vi "PID control.vi"(4 "auto? (F)":bool, 5 "dt (s)":dbl, 6 "PID gains":T1={"proportional gain (Kc)"=1.0, "integral time (Ti, min)"=0.01, "derivative time (Td, min)"=0.0} {"derivative time (Td, min)" format="%#.6g"; "integral time (Ti, min)" format="%#.6g"; "proportional gain (Kc)" format="%#.6g"}, 7 "Waveform Function (0: Sine)":u16(ring)=1 items=["Sine", "Square", "Ramp", "DC", "Pulse", "Arb"], 8 "error in (no error)":errorcluster, 9 "Frequency (Hz)":dbl=1000.0 min=1e-06 max=160000000.0 step=1.0 format="%#.6g", 10 "Amplitude setpoint (V)":dbl=1.0 min=0.001 max=20.0 step=1.0 format="%#.3f", 11 "VISA resource name":refnum<visa-resource-name>) -> (0 "error out":errorcluster, 3 "VISA resource name out":refnum<visa-resource-name>)   [LabVIEW 2017]
uses:
  <vilib>/addons/control/pid/autopid.llb/PID autotuning parameters (adv).ctl
  <vilib>/DAQmx/read.llb/DAQmx Read (Analog Wfm 1Chan NSamp).vi
  <vilib>/Analysis/baseanly.llb/Mean (DBL).vi
  <vilib>/DAQmx/miscellaneous.llb/DAQmx Fill In Error Info.vi
  <instrlib>/Siglent SDG 1000 5000 800 Series/Siglent SDG 1000 5000 800 Series.lvlib
  <vilib>/Analysis/NI_AALBase.lvlib
  <vilib>/addons/control/pid/NI_PID_autopid.lvlib
panel:
  in  "stop":bool
  out "Measured amplitude (V)":dbl format="%0.2f"
  out "tuning completed?":bool
  out "Control amplitude (V)":dbl
  in  "output range":cluster{"output high":dbl, "output low":dbl}={"output high"=10.0, "output low"=0.0}
  out "tuned PID gains":T1={"proportional gain (Kc)"=1.0, "integral time (Ti, min)"=0.01, "derivative time (Td, min)"=0.0} {"derivative time (Td, min)" format="%#.6g"; "integral time (Ti, min)" format="%#.6g"; "proportional gain (Kc)" format="%#.6g"}
  in  "autotuning parameters":T2={"technique"=2, "type of controller"=1, "control specification"=0, "amplitude"=1.0} {"amplitude" format="%.2f"; "control specification" items=["normal", "fast", "slow"]; "type of controller" items=["P", "PI", "PID"]; "technique" items=["Step Open Loop", "Step Closed Loop", "Relay", "PID Relay"]}
  in  "reinitialize? (F)":bool
  in  "autotune? (F)":bool
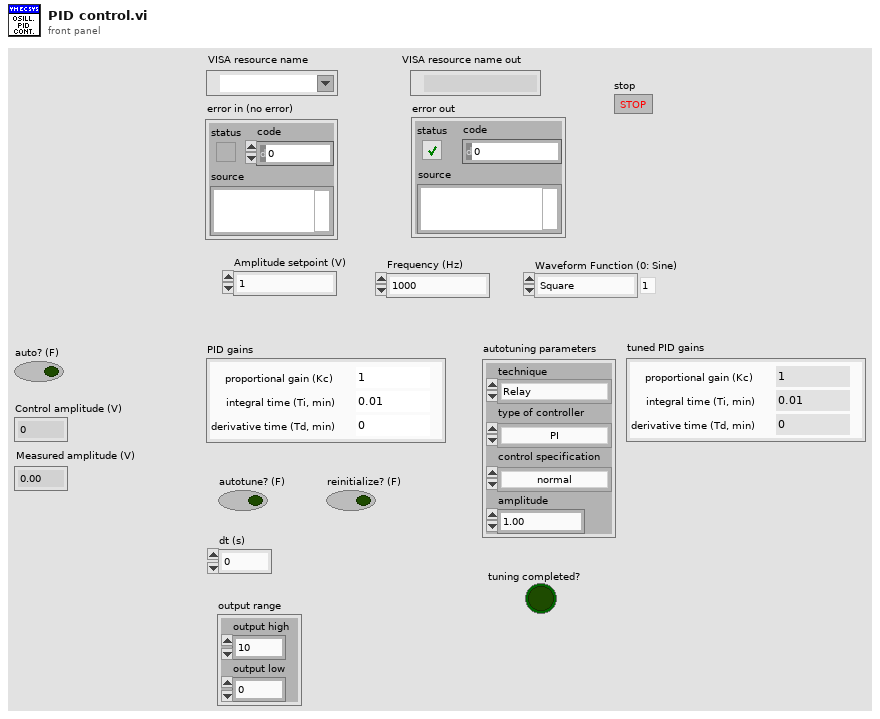
[diagram p1: front panel]
types:
  T1 = cluster{"proportional gain (Kc)":dbl, "integral time (Ti, min)":dbl, "derivative time (Td, min)":dbl}
  T2 = typedef "NI_PID_autopid.lvlib/PID autotuning parameters (adv).ctl" = cluster{"technique":u16, "type of controller":u16, "control specification":u16, "amplitude":dbl}
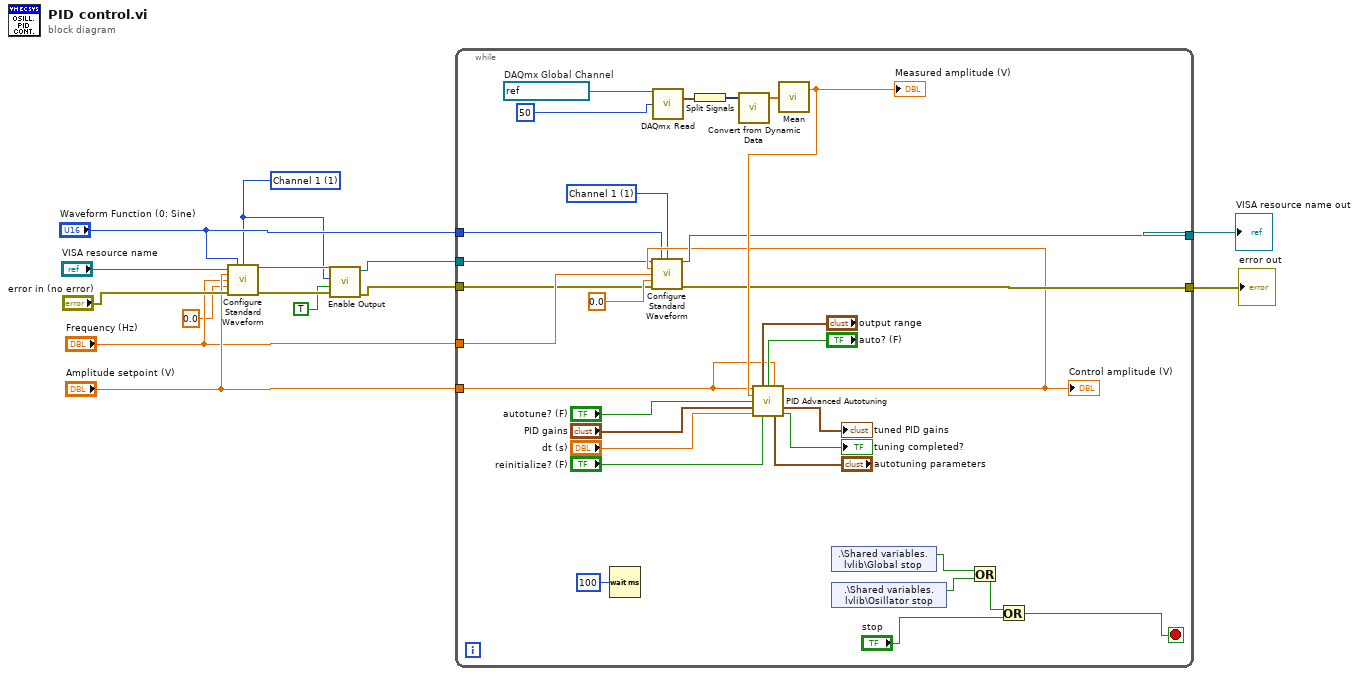
[diagram p0: block diagram]
diagram:
  w2 = 1 items=["Channel 1"=1, "Channel 2"=2] ("Channel (1:Channel 1)")
  n1 = call <instrlib>:"Configure Standard Waveform.vi"("VISA resource name"="VISA resource name", "Waveform Function (0: Sine)"="Waveform Function (0: Sine)", "Channel (1:Channel 1)"=w2, "Amplitude (1.0 Vpp)"="Amplitude setpoint (V)", "Frequency (1000 Hz)"="Frequency (Hz)", "DC Offset (0.00 V)"=0.0, "error in (no error)"="error in (no error)") -> ("VISA resource name out"=w9:refnum<visa-resource-name>, "error out"=w10:errorcluster)  [unwired: 7 in]
  n2 = call <instrlib>:"Enable Output.vi"("error in (no error)"=w10, "Enable Output (T: Enable)"=TRUE, "Channel (1:Channel 1)"=w2, "VISA resource name"=w9) -> ("error out"=w7:errorcluster, "VISA resource name out"=w8:refnum<visa-resource-name>)  [unwired: 6 in]
  n3 = while {
    tunnel: "Frequency (Hz)" -> [w40]
    tunnel: "Amplitude setpoint (V)" -> [w25]
    tunnel: [w31] -> w14
    tunnel: [w30] -> w13
    tunnel: "Waveform Function (0: Sine)" -> [w18]
    tunnel: w8 -> [w17]
    tunnel: w7 -> [w16]
    stop <- w19 stop-if-true
    w15 = 1 items=["Channel 1"=1, "Channel 2"=2] ("Channel (1:Channel 1)")
    w45 = refnum<k21> "AC voltage"  # DAQmx Global Channel
    n4 = Wait (ms)(milliseconds to wait=u32 100) -> ()  [unwired: 1 out]
    n5 = call-poly <vilib>:"DAQmx Read.vi"("task/channels in"=w45, "number of samples per channel"=50) -> ("data"=w44:waveform(dbl))  [unwired: 11 in, 2 out]
    n6 = Split Signals(w44) -> (w43:dynamicdata)  [unwired: 1 in]
    n7 = call "Convert from Dynamic Data"("Dynamic Data Type"=w43) -> ("Array"=w42:dbl[])  [unwired: 3 in]
    n8 = call-poly <vilib>:"Mean.vi"("X"=w42) -> ("mean"=w38:dbl)  [unwired: 1 out]
    "Measured amplitude (V)" <- w38
    n9 = call <vilib>:"PID Advanced Autotuning.vi"("setpoint"=w25, "output range"="output range", "auto? (F)"="auto? (F)", "manual control"=w25, "process variable"=w38, "autotune? (F)"="autotune? (F)", "PID gains"="PID gains", "dt (s)"="dt (s)", "reinitialize? (F)"="reinitialize? (F)", "autotuning parameters"="autotuning parameters") -> ("output"=w27:dbl, "tuned PID gains"=→"tuned PID gains":T1, "tuning completed?"=→"tuning completed?":bool)  [unwired: 3 in]
    "Control amplitude (V)" <- w27
    n10 = call <instrlib>:"Configure Standard Waveform.vi"("VISA resource name"=w17, "Waveform Function (0: Sine)"=w18, "Channel (1:Channel 1)"=w15, "Amplitude (1.0 Vpp)"=w27, "Frequency (1000 Hz)"=w40, "DC Offset (0.00 V)"=0.0, "error in (no error)"=w16) -> ("VISA resource name out"=w30:refnum<visa-resource-name>, "error out"=w31:errorcluster)  [unwired: 7 in]
    n11 = shared-variable ".\\Shared variables.lvlib\\Global stop"() -> (w23:bool)  [unwired: 1 in, 1 out]
    n12 = shared-variable ".\\Shared variables.lvlib\\Osillator stop"() -> (w22:bool)  [unwired: 1 in, 1 out]
    n13 = Or(x=w23, y=w22) -> (x .or. y?=w20:bool)
    n14 = Or(x=w20, y="stop") -> (x .or. y?=w19:bool)
  }
  "error out" <- w14
  "VISA resource name out" <- w13
